vi "Manual Intake Mode.vi"(6 "Current Encoder Position":dbl) -> (1 "Rollers Active?":bool, 2 "Arm Power":dbl, 3 "Intake Power":dbl)   [LabVIEW 2015]
uses:
  Robot Global Data.vi
  <vilib>/addons/control/pid/pid.llb/PID (DBL).vi
  <vilib>/addons/control/pid/NI_PID_pid.lvlib
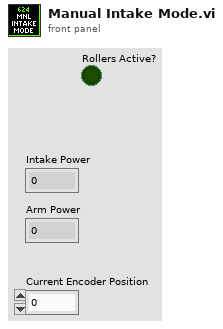
[diagram p1: front panel]
types:
  T1 = typedef "Dashboard Control Data.ctl" = cluster{"Shooter Presets":T2, "Encoder Control":T4, "Steer PID output":cluster{"output high":dbl, "output low":dbl}, " Steer PID gains":cluster{"proportional gain (Kc)":dbl, "integral time (Ti, min)":dbl, "derivative time (Td, min)":dbl}, "Drivetrain Settings":T5, "Vision Packet":T6, "Dashboard Drivetrain Command":T7, "Info/Command Cluster":T9, "Ball Vision Packet":T10, "Intake Presets":T12, "Intake Encoder Control":T14, "Climb Presets":T15, "Ultrasonic Limit":dbl, "Roll Limit":dbl, "Pitch Limit":dbl, "Goal Output Range":cluster{"output high":dbl, "output low":dbl}}
  T2 = typedef "Shooter Presets.ctl" = cluster{"Batter Shot":T3, "Deep Middle Shot":T3, "Manual Shot":T3, "Left Ticks Per Rotation":dbl, "Right Ticks Per Rotation":dbl, "Low Bar Shot":T3, "Shooter RPM Tolerance":dbl, "IIR Filter Power":dbl, "Trigger Power":dbl, "Fire from Load Delay":i32, "Angle Pot M":dbl, "Angle Pot B":dbl, "Shooter Length":dbl, "String Pot Dist":dbl, "Angle PID gains":cluster{"proportional gain (Kc)":dbl, "integral time (Ti, min)":dbl, "derivative time (Td, min)":dbl}, "Angle Motor Output":cluster{"output high":dbl, "output low":dbl}, "Shooter Angle Tolerance":dbl, "Vision Shoot x^2":dbl, "Vision Shoot x":dbl, "Dist from Axis Cam to Pivot":dbl, "High Goal Center Height":dbl, "Feed Forward Max Accel":dbl, "Feed Forward Kv":dbl, "Backwards Trigger":dbl, "Shot Finish Delay (ms)":dbl, "Angle Max Current":dbl, "Angle Current Trip Time":dbl, "Shooter Intake Angle":dbl, "Vision Shoot c":dbl, "Reset?":bool, "Servo Release Delay":dbl, "Servo Idle Angle":i32, "Servo Hold Angle":i32, "Angle Pot x^2":dbl, "Angle Pot x":dbl, "Angle Pot c":dbl}
  T3 = typedef "Shot Presets.ctl" = cluster{"Left Wheel RPM":dbl, "Right Wheel RPM":dbl, "Angle":dbl}
  T4 = typedef "Encoder Control.ctl" = cluster{"Right Tick Constant":dbl, "Left Tick Constant":dbl, "Reset?":bool, "Y Dist":cluster{"PID gains":cluster{"proportional gain (Kc)":dbl, "integral time (Ti, min)":dbl, "derivative time (Td, min)":dbl}}, "Y Stop Thresh":dbl, "Y Stop Speed":dbl}
  T5 = typedef "Drivetrain Settings.ctl" = cluster{"Gyro Tolerance":dbl, "Throttle Ramp (ms)":dbl, "Angular rate compensation":bool, "Throttle to Rate Scale":dbl, "Rate compensation gain":dbl, "Kv":dbl, "Ka":dbl, "Feed Forward P":dbl, "Feed Forward D":dbl, "Goal Vision PID gains":cluster{"proportional gain (Kc)":dbl, "integral time (Ti, min)":dbl, "derivative time (Td, min)":dbl}, "Goal Detection Window":dbl}
  T6 = typedef "Goal Vision Packet.ctl" = cluster{"Distance":dbl, "Center X":dbl, "Center Y":dbl, "Found Target?":bool}
  T7 = typedef "Dashboard Drivetrain Command.ctl" = cluster{"Drivetrain Vision":T8}
  T8 = typedef "Drivetrain Vision.ctl" = cluster{"Goal Window":dbl, "Ball Window":dbl}
  T9 = typedef "Ball Tracking Command Cluster.ctl" = cluster{"Distance to Ball":dbl, "Desired Angle":dbl, "Command":enum16{"Turn to Ball", "Turn to Angle", "Get Distance"}, "Pixels from Center":dbl}
  T10 = typedef "Ball Vision Packet.ctl" = cluster{"Ball Detected?":bool, "Distance to Ball":dbl, "Desired Angle":dbl, "Pixels from Center":dbl, "Tracking mode":T11}
  T11 = typedef "Tracking Mode.ctl" = enum16{"Turn to Ball", "Turn to Angle"}
  T12 = typedef "Intake Presets.ctl" = cluster{"Intake Speed":dbl, "Outake Speed":dbl, "Low Height":dbl, "Half Height":dbl, "Full Height":dbl, "Angle Speed":dbl, "Fast Angle":dbl, "Encoder Scale":dbl, "Load Height":dbl, "Output Range":T13, "Rotation Power Max/Min":dbl, "MaxCurrent":dbl, "Intake Trip Time":dbl, "Idle Height":dbl, "Max Height":dbl, "Reset Encoders?":bool, "PID gains":cluster{"proportional gain (Kc)":dbl, "integral time (Ti, min)":dbl, "derivative time (Td, min)":dbl}}
  T13 = typedef "Drivetrain Output Range.ctl" = cluster{"output high":dbl, "output low":dbl}
  T14 = typedef "IntakeEcoderControl.ctl" = cluster{"Arm Tick Constant":dbl, "Reset?":bool, "Y Dist":cluster{"PID gains":cluster{"proportional gain (Kc)":dbl, "integral time (Ti, min)":dbl, "derivative time (Td, min)":dbl}}, "Y Stop Thresh":dbl, "Y Stop Speed":dbl}
  T15 = typedef "Climb Presets.ctl" = cluster{"Pull Power":dbl, "Unpin Power":dbl, "Time to Hold":dbl}
  T16 = typedef "Manual Intake Commands.ctl" = cluster{"Intake":bool, "Eject":bool, "Arm Angle":dbl, "Intake Override Speed":dbl, "Arm Override Speed":dbl, "Arm Speed":dbl, "Override Intake":bool, "Override Eject":bool, "Eject Override Speed":dbl, "Arm":bool, "Override Arm":bool, "Override Angle":bool}
  T17 = cluster{"proportional gain (Kc)":dbl, "integral time (Ti, min)":dbl, "derivative time (Td, min)":dbl}
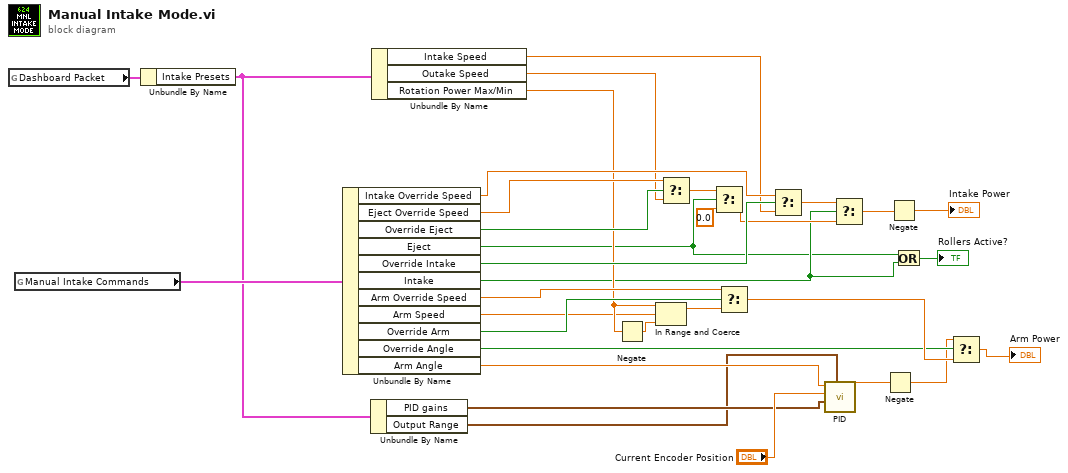
[diagram p0: block diagram]
diagram:
  n1 = global read "Robot Global Data.vi" "Dashboard Packet"() -> (w24:T1)
  n2 = global read "Robot Global Data.vi" "Manual Intake Commands"() -> (w21:T16)
  n3 = Unbundle By Name(w24) -> ("Intake Presets"=w8:T12)
  n4 = Unbundle By Name(w21) -> ("Intake Override Speed"=w27:dbl, "Eject Override Speed"=w33:dbl, "Override Eject"=w32:bool, "Eject"=w12:bool, "Override Intake"=w29:bool, "Intake"=w13:bool, "Arm Override Speed"=w25:dbl, "Arm Speed"=w17:dbl, "Override Arm"=w20:bool, "Override Angle"=w4:bool, "Arm Angle"=w10:dbl)
  n5 = Unbundle By Name(w8) -> ("PID gains"=w7:T17, "Output Range"=w6:T13)
  n6 = Unbundle By Name(w8) -> ("Intake Speed"=w23:dbl, "Outake Speed"=w22:dbl, "Rotation Power Max/Min"=w19:dbl)
  n7 = Negate(x=w19) -> (-x=w18:dbl)
  n8 = In Range and Coerce(upper limit=w19, x=w17, lower limit=w18) -> (coerced(x)=w16:dbl)  [unwired: 1 out]
  n9 = Select(t=w33, s=w32, f=w22) -> (s? t:f=w31:dbl)
  n10 = Select(t=w31, s=w12, f=0.0) -> (s? t:f=w26:dbl)
  n11 = Select(t=w25, s=w20, f=w16) -> (s? t:f=w5:dbl)
  n12 = Select(t=w27, s=w29, f=w23) -> (s? t:f=w30:dbl)
  n13 = call-poly <vilib>:"PID.vi"("output range"=w6, "PID gains"=w7, "process variable"="Current Encoder Position", "setpoint"=w10) -> ("output"=w3:dbl)  [unwired: 6 in, 1 out]
  n14 = Select(t=w30, s=w13, f=w26) -> (s? t:f=w15:dbl)
  n15 = Negate(x=w3) -> (-x=w2:dbl)
  n16 = Negate(x=w15) -> (-x=→"Intake Power":dbl)
  n17 = Or(x=w12, y=w13) -> (x .or. y?=→"Rollers Active?":bool)
  n18 = Select(t=w2, s=w4, f=w5) -> (s? t:f=→"Arm Power":dbl)
